vi "Program Name.vi"() -> (3 "Program Name":string)   [LabVIEW 2018, in "Config Module.lvlib"]
uses:
  Config Module.lvlib
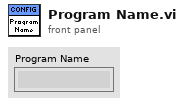
[diagram p1: front panel]
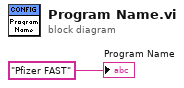
[diagram p0: block diagram]
diagram:
  "Program Name" <- "Pfizer FAST" ("name or relative path")
